vi "Insight_Instantaneous_Phase.vi"(8 "error in (no error)":errorcluster, 10 "X-axis":dbl[](array[numeric]), 11 "Data":dbl[](array[numeric])) -> (0 "error out":errorcluster, 1 "Phase Residuals (rad)":dbl[](array[numeric]), 2 "Unwrapped Phase (rad)":dbl[](array[numeric]), 3 "Envelope":dbl[](array[numeric]))   [LabVIEW 2010]
uses:
  <vilib>/Analysis/NI_AALPro.lvlib
  <vilib>/Analysis/6fits.llb/Curve Fitting Criteria.ctl
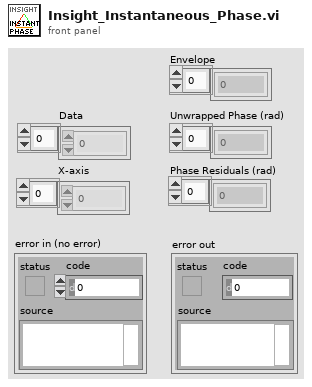
[diagram p1: front panel]
types:
  T1 = typedef "NI_AALPro.lvlib/Curve Fitting Criteria.ctl" = u16
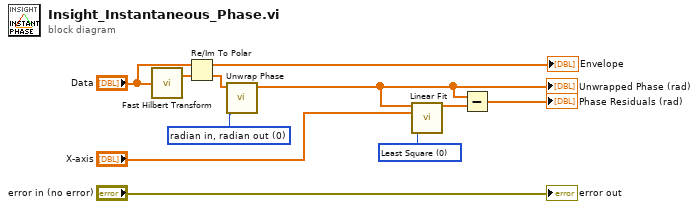
[diagram p0: block diagram]
diagram:
  w10 = T1 0 items=["Least Square", "Least Absolute Residual", "Bisquare"] ("method")
  w11 = 0 items=["radian in, radian out", "radian in, degree out", "degree in, degree out", "degree in, radian out"] ("phase unit")
  n1 = call <vilib>:"Fast Hilbert Transform.vi"("X"="Data") -> ("Hilbert{X}"=w5:dbl[])  [unwired: 1 out]
  n2 = Re/Im To Polar(2:w5, 3:"Data") -> (0:w3:dbl[], 1:→"Envelope":dbl[])
  n3 = call <vilib>:"Unwrap Phase.vi"("phase unit"=w11, "Phase"=w3) -> ("Unwrapped Phase"=w8:dbl[])  [unwired: 8 in, 1 out]
  "Unwrapped Phase (rad)" <- w8
  n4 = call <vilib>:"Linear Fit.vi"("Y"=w8, "X"="X-axis", "method"=w10) -> ("Best Linear Fit"=w9:dbl[])  [unwired: 8 in, 4 out]
  n5 = Subtract(x=w8, y=w9) -> (x-y=→"Phase Residuals (rad)":dbl[])
  "error out" <- "error in (no error)"
